vi "Update_CW.vi"(7 "channel name (\"1\")":string="1", 8 "error in (no error)":errorcluster {"code" format="%.0x"}, 9 "CM cluster":T1={"Frequency (Hz)"=80000000.0, "Amplitude (V)"=0.2, "Phase (°)"=0.0, "Offset (Volt)"=0.0, "waveform (1: Sine)"=1, "output mode"=0, "Modulation Waveform (1: Sine)"=1} {"Modulation Waveform (1: Sine)" items=["Sine"=1, "Square"=2, "Triangle"=3, "Ramp Up"=4, "Ramp Down"=5, "Noise"=100, "Arbitrary User1"=200, "Arbitrary User2"=201, "Arbitrary User3"=202, "Arbitrary User4"=203, "Edit Memory"=204]; "output mode" items=["Standard Function", "Arbitrary Waveform"]; "waveform (1: Sine)" items=["Sine"=1, "Square"=2, "Pulse"=1002, "Ramp"=1001, "Noise"=1003, "DC"=6, "Sin(x)/x"=1004, "Gaussian"=1005, "Lorentz"=1006, "Exponential Rise"=1007, "Exponential Decay"=1008, "Haversine"=1009]}, 11 "resource name":refnum<k15>) -> (0 "error out":errorcluster {"code" format="%.0x"}, 1 "output cluster":T2, 3 "instrument handle out":refnum<k15>)   [LabVIEW 2015, in "MyToolsFunction.lvlib"]
uses:
  ICcamera/MyToolsFunction.lvlib
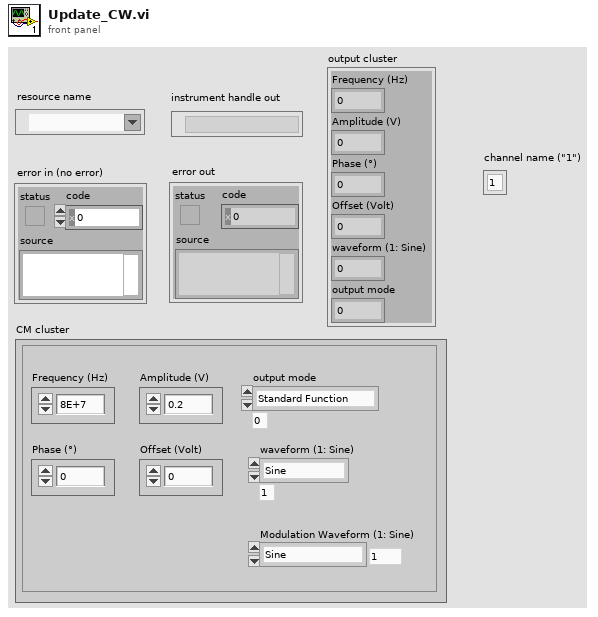
[diagram p1: front panel]
types:
  T1 = cluster{"Frequency (Hz)":dbl, "Amplitude (V)":dbl, "Phase (°)":dbl, "Offset (Volt)":dbl, "waveform (1: Sine)":i32, "output mode":i32, "Modulation Waveform (1: Sine)":i32}
  T2 = cluster{"Frequency (Hz)":dbl, "Amplitude (V)":dbl, "Phase (°)":dbl, "Offset (Volt)":dbl, "waveform (1: Sine)":i32, "output mode":i32}
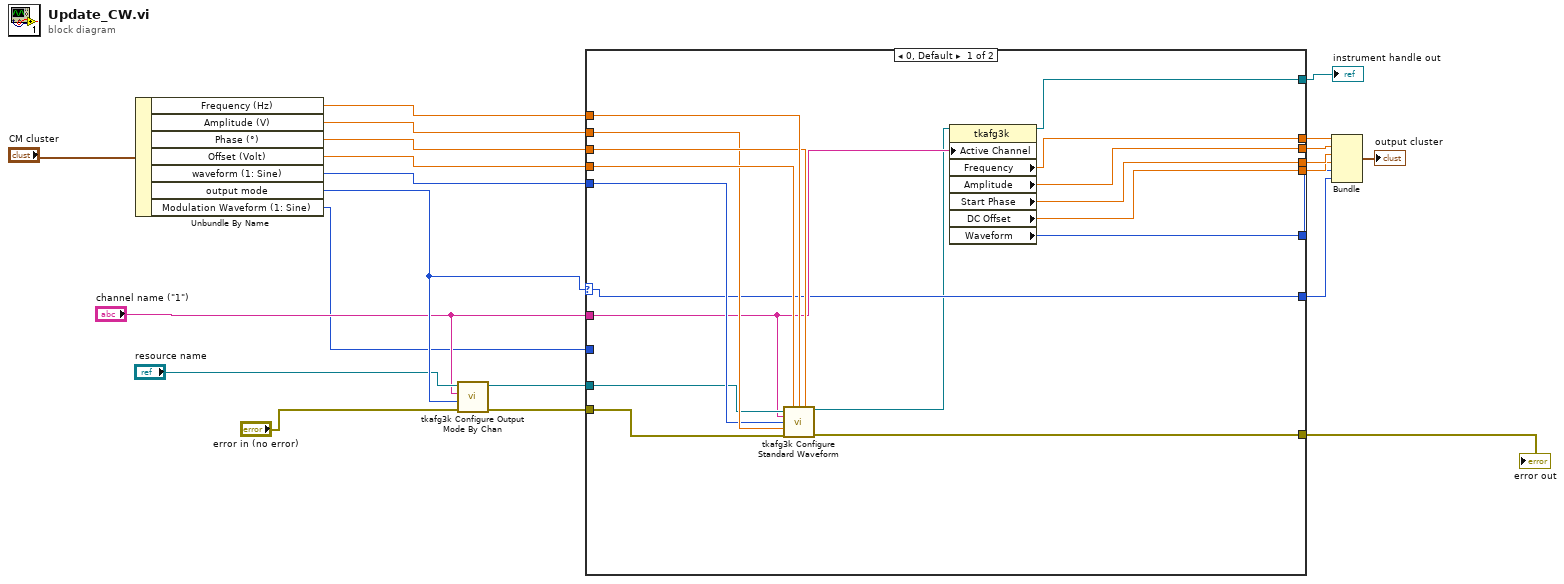
[diagram p0: block diagram]
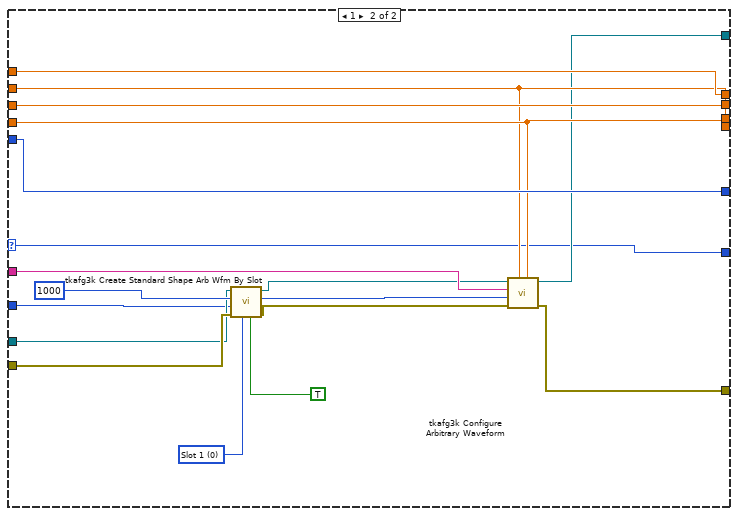
[diagram p2: hidden frame]
diagram:
  n1 = Unbundle By Name("CM cluster") -> ("Frequency (Hz)"=w21:dbl, "Amplitude (V)"=w19:dbl, "Phase (°)"=w20:dbl, "Offset (Volt)"=w22:dbl, "waveform (1: Sine)"=w18:i32, "output mode"=w6:i32, "Modulation Waveform (1: Sine)"=w1:i32)
  n2 = call <instrlib>:"tkafg3k Configure Output Mode By Chan.vi"("error in (no error)"="error in (no error)", "Output Mode (0: Standard Function)"=w6, "Channel Name (\"1\")"="channel name (\"1\")", "instrument handle"="resource name") -> ("error out"=w8:errorcluster, "instrument handle out"=w5:refnum<k15>)  [unwired: 6 in]
  n3 = case shown="0, Default" w6 {
    selector: w6 -> [w25 w49]
    tunnel: w22 -> [w39 w54]
    tunnel: w21 -> [w38 w55]
    tunnel: w20 -> [w37 w57]
    tunnel: w19 -> [w36 w53]
    tunnel: w18 -> [w35 w56]
    tunnel: w5 -> [w34 w45]
    tunnel: w8 -> [w33 w48]
    tunnel: [w32 w50] -> w17
    tunnel: [w23 w51] -> w16
    tunnel: "channel name (\"1\")" -> [w31 w52]
    tunnel: [w30 w55] -> w15
    tunnel: [w29 w53] -> w14
    tunnel: [w28 w57] -> w13
    tunnel: [w27 w54] -> w12
    tunnel: [w26 w56] -> w11
    tunnel: [w25 w49] -> w10
    tunnel: w1 -> [_ w40]
    frame 0, Default {
      n4 = call <instrlib>:"tkafg3k Configure Standard Waveform.vi"("instrument handle"=w34, "dc offset (0.00)"=w39, "frequency (1000000)"=w38, "start phase (0.00)"=w37, "channel name (\"1\")"=w31, "waveform (1: Sine)"=w35, "amplitude (1)"=w36, "error in (no error)"=w33) -> ("instrument handle out"=w24:refnum<k15>, "error out"=w32:errorcluster)  [unwired: 6 in]
      n5 = property class="tkafg3k"(reference=w24, "Active Channel"=w31) -> (reference out=w23:refnum<k15>, "Frequency"=w30:dbl, "Amplitude"=w29:dbl, "Start Phase"=w28:dbl, "DC Offset"=w27:dbl, "Waveform"=w26:i32)  [unwired: 1 in, 1 out]
    }
    frame 1 {
      w44 = 0 items=["Slot 1", "Slot 2", "Slot 3", "Slot 4"] ("slot (0: Slot 1)")
      n6 = call <instrlib>:"tkafg3k Create Standard Shape Arb Wfm By Slot.vi"("overwrite (False)"=TRUE, "slot (0: Slot 1)"=w44, "error in (no error)"=w48, "Waveform Type (SINE)"=w40, "Waveform Size (1000)"=1000, "instrument handle"=w45) -> ("error out"=w47:errorcluster, "Waveform Handle"=w42:i32, "instrument handle out"=w41:refnum<k15>)  [unwired: 3 in]
      n7 = call <instrlib>:"tkafg3k Configure Arbitrary Waveform.vi"("offset (0.00)"=w54, "gain (0.5)"=w53, "error in (no error)"=w47, "waveform handle"=w42, "channel name (\"1\")"=w52, "instrument handle"=w41) -> ("error out"=w50:errorcluster, "instrument handle out"=w51:refnum<k15>)  [unwired: 4 in]
    }
  }
  "error out" <- w17
  "instrument handle out" <- w16
  n8 = Bundle("Frequency (Hz)"=w15, "Amplitude (V)"=w14, "Phase (°)"=w13, "Offset (Volt)"=w12, "waveform (1: Sine)"=w11, "output mode"=w10) -> (→"output cluster":T2)  [unwired: 1 in]
